vi "GET.vi"(6 "timeout (10000)":i32=10000, 7 "output file":path=path "", 8 "error in (no error)":errorcluster, 10 "url":string, 11 "HTTP Client reqwest in":refnum<class "HTTP Client reqwest.lvclass">) -> (0 "error out":errorcluster, 1 "body":string, 2 "headers":string, 3 "HTTP Client reqwest out":refnum<class "HTTP Client reqwest.lvclass">, 4 "status code":u32)   [LabVIEW 2020, in "HTTP Client reqwest.lvclass"]
uses:
  HTTP Client reqwest.lvclass
  HTTP Client reqwest.lvclass/HTTP Client reqwest.ctl
  Types/http_method_enum.ctl
  RequestBuilder/RequestBuilder.lvclass
  Client/Client.lvclass
  reqwest.lvlib
  Request/Request.lvclass
  Headers/Headers.lvclass
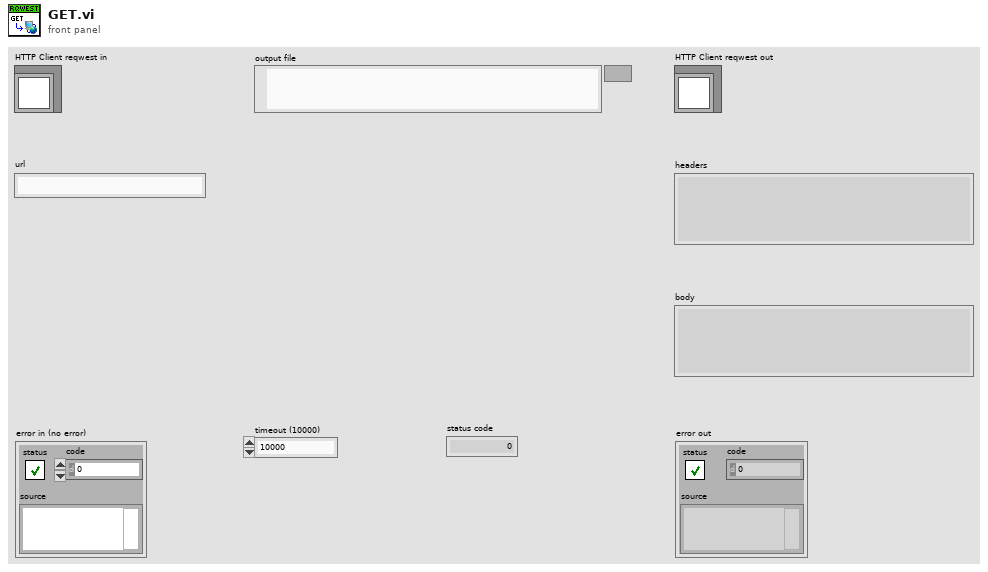
[diagram p1: front panel]
types:
  T1 = typedef "reqwest.lvlib/http_method_enum.ctl" = enum8{"<select>", "GET", "POST", "PUT", "DELETE", "HEAD", "OPTIONS", "CONNECT", "PATCH", "TRACE"}
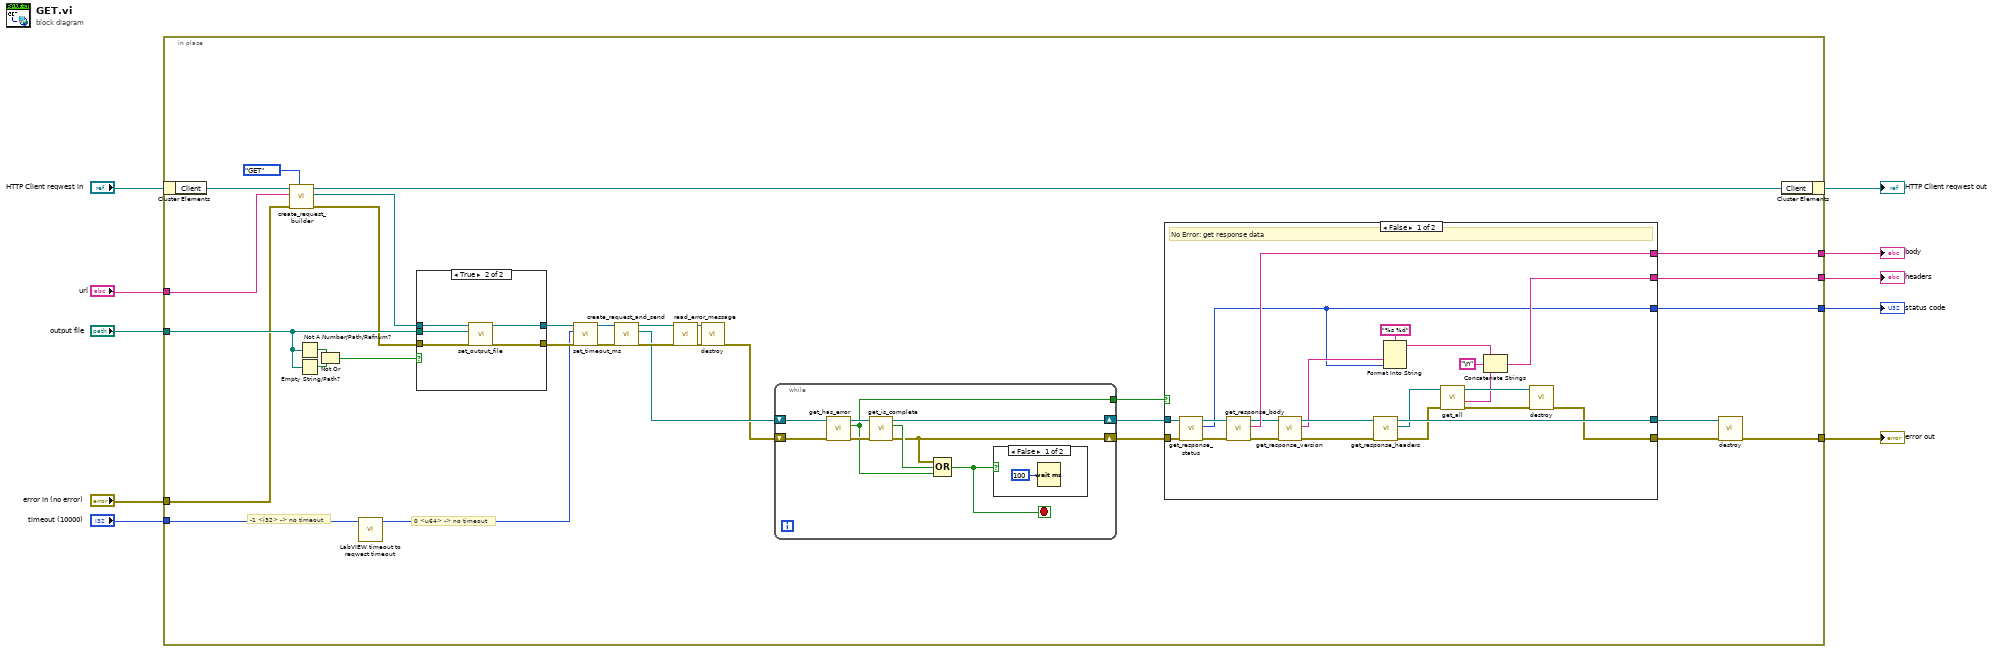
[diagram p0: block diagram]
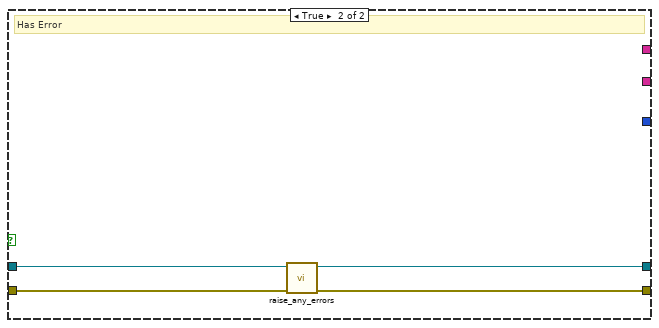
[diagram p2: hidden frame]
diagram:
  n1 = in-place {
    in-place-border: "url" -> [w40]
    in-place-border: "output file" -> [w35]
    in-place-border: "error in (no error)" -> [w34]
    in-place-border: [w22] -> w5
    in-place-border: [w20] -> w4
    in-place-border: [w19] -> w3
    in-place-border: [w12] -> w2
    in-place-border: "timeout (10000)" -> [w14]
    # "0 <u64> -> no timeout"
    # "-1 <i32> -> no timeout"
    n2 = in-place-cluster #1("HTTP Client reqwest in") -> ("Client"=w41:refnum<class "Client.lvclass">)
    n3 = call "create_request_builder.vi"("HTTP Method"=http_method_enum."GET", "error in (no error)"=w34, "url"=w40, "Client in"=w41) -> ("error out"=w33:errorcluster, "RequestBuilder out"=w36:refnum<class "RequestBuilder.lvclass">, "Client out"=w21:refnum<class "Client.lvclass">)  [unwired: 5 in]
    n4 = Not A Number/Path/Refnum?(number/path/refnum=w35) -> (NaN/Path/Refnum?=w38:bool)
    n5 = Empty String/Path?(string/path=w35) -> (empty?=w39:bool)
    n6 = Not Or(1:w39, 2:w38) -> (0:w37:bool)
    n7 = call "LabVIEW timeout to reqwest timeout.vi"("-1 -> no timeout"=w14) -> ("0 -> no timeout"=w13:u64)  [unwired: 10 in]
    n8 = case shown="True" w37 {
      tunnel: w36 -> [w69 w75]
      tunnel: w35 -> [_ w74]
      tunnel: [w69 w73] -> w18
      tunnel: w33 -> [w70 w72]
      tunnel: [w70 w71] -> w16
      frame False {
      }
      frame True {
        n9 = call "set_output_file.vi"("error in (no error)"=w72, "output_file"=w74, "obj in"=w75) -> ("error out"=w71:errorcluster, "obj out"=w73:refnum<class "RequestBuilder.lvclass">)  [unwired: 6 in, 1 out]
      }
    }
    n10 = call "set_timeout_ms.vi"("error in (no error)"=w16, "timeout_ms"=w13, "obj in"=w18) -> ("error out"=w15:errorcluster, "obj out"=w17:refnum<class "RequestBuilder.lvclass">)  [unwired: 6 in, 1 out]
    n11 = call "create_request_and_send.vi"("error in"=w15, "obj in"=w17) -> ("error out"=w32:errorcluster, "request"=w28:refnum<class "Request.lvclass">, "obj out"=w31:refnum<class "RequestBuilder.lvclass">)  [unwired: 7 in]
    n12 = call "read_error_message.vi"("error in (no error)"=w32, "RequestBuilder in"=w31) -> ("error out"=w30:errorcluster, "RequestBuilder in"=w29:refnum<class "RequestBuilder.lvclass">)  [unwired: 7 in, 1 out]
    n13 = call "destroy.vi"("error in"=w30, "RequestBuilder in"=w29) -> ("error out"=w27:errorcluster)  [unwired: 8 in, 1 out]
    n14 = while {
      shift-right: [w79] -> w23
      shift-left: w28 -> [w83]
      shift-right: [w78] -> w24
      shift-left: w27 -> [w82]
      tunnel: [w76] -> w11
      stop <- w77 stop-if-true
      n15 = call "get_has_error.vi"("error in (no error)"=w82, "Request in"=w83) -> ("error out"=w80:errorcluster, "has_error"=w76:bool, "Request out"=w81:refnum<class "Request.lvclass">)  [unwired: 7 in]
      n16 = call "get_is_complete.vi"("error in (no error)"=w80, "Request in"=w81) -> ("error out"=w78:errorcluster, "is_complete"=w84:bool, "Request out"=w79:refnum<class "Request.lvclass">)  [unwired: 7 in]
      n17 = Compound Arithmetic op=OR(w78, w84, w76) -> (w77:bool)
      n18 = case shown="False" w77 {
        frame False {
          n19 = Wait (ms)(milliseconds to wait=u32 100) -> ()  [unwired: 1 out]
        }
        frame True {
        }
      }
    }
    n20 = case shown="False" w11 {
      tunnel: [w64 w67] -> w26
      tunnel: [w59 w68] -> w25
      tunnel: [w58 _] -> w20
      tunnel: [w52 _] -> w19
      tunnel: w23 -> [w47 w65]
      tunnel: w24 -> [w45 w66]
      tunnel: [w43 _] -> w12
      frame False {
        # "No Error: get response data"
        n21 = call "get_response_status.vi"("error in (no error)"=w45, "Request in"=w47) -> ("error out"=w44:errorcluster, "status_code"=w43:u16, "Request out"=w46:refnum<class "Request.lvclass">)  [unwired: 7 in]
        n22 = call "get_response_body.vi"("error in (no error)"=w44, "Request in"=w46) -> ("error out"=w55:errorcluster, "string_value"=w58:string, "Request in"=w57:refnum<class "Request.lvclass">)  [unwired: 7 in]
        n23 = call "get_response_version.vi"("error in (no error)"=w55, "Request in"=w57) -> ("error out"=w54:errorcluster, "response_version"=w49:string, "Request in"=w56:refnum<class "Request.lvclass">)  [unwired: 7 in]
        n24 = call "get_response_headers.vi"("error in (no error)"=w54, "Request in"=w56) -> ("error out"=w62:errorcluster, "response_headers"=w63:refnum<class "Headers.lvclass">, "Request in"=w64:refnum<class "Request.lvclass">)  [unwired: 7 in]
        n25 = Format Into String(format string="%s %d", w49, w43) -> (resulting string=w48:string)  [unwired: 2 in, 1 out]
        n26 = call "get_all.vi"("error in (no error)"=w62, "Headers in"=w63) -> ("error out"=w60:errorcluster, "headers"=w53:string, "Headers in"=w61:refnum<class "Headers.lvclass">)  [unwired: 6 in, 1 out]
        n27 = Concatenate Strings(w48, "\n" ("string"), w53) -> (w52:string)
        n28 = call "destroy.vi"("error in (no error)"=w60, "Headers in"=w61) -> ("error out"=w59:errorcluster)  [unwired: 9 in]
      }
      frame True {
        # "Has Error"
        n29 = call "raise_any_errors.vi"("error in (no error)"=w66, "Request in"=w65) -> ("error out"=w68:errorcluster, "Request out"=w67:refnum<class "Request.lvclass">)  [unwired: 8 in]
      }
    }
    n30 = call "destroy.vi"("error in (no error)"=w25, "Request in"=w26) -> ("error out"=w22:errorcluster)  [unwired: 8 in, 1 out]
    n31 = in-place-cluster #1("Client"=w21) -> (→"HTTP Client reqwest out":refnum<class "HTTP Client reqwest.lvclass">)
  }
  "error out" <- w5
  "headers" <- w3
  "body" <- w4
  "status code" <- w2
